vi "isBrushSet.vi"(8 "Error In":errorcluster, 9 "colorRole":T1 items=["WindowText", "Button", "Light", "Midlight", "Dark", "Mid", "Text", "BrightText", "ButtonText", "Base", "Window", "Shadow", "Highlight", "HighlightedText", "Link", "LinkVisited", "AlternateBase", "NoRole", "ToolTipBase", "ToolTipText", "PlaceholderText"], 10 "colorGroup":T2 items=["Active"=0, "Disabled"=1, "Inactive"=2, "All"=5], 11 "QPalette In":refnum<class "QPalette.lvclass">) -> (0 "Error Out":errorcluster, 2 "Value":bool, 3 "QPalette Out":refnum<class "QPalette.lvclass">)   [LabVIEW 2014, in "QPalette.lvclass"]
doc: "LabVIEW-specific documentation is not yet available. See <b>https://doc.qt.io/qt-5/qpalette.html#isBrushSet</b>"
uses:
  QPalette.lvclass
  ColorGroup.ctl
  ColorRole.ctl
  LQ Core/LQSerialData/LQSerialData.lvclass/LQSerialData.ctl
  LQ Core/LQ Core.lvlib
  LQ Core/LQSerialData/LQSerialData.lvclass
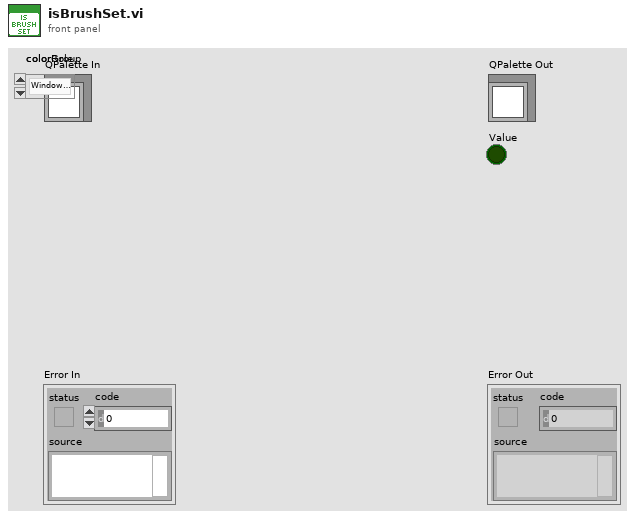
[diagram p1: front panel]
types:
  T1 = typedef "QPalette.lvclass/ColorRole.ctl" = i32
  T2 = typedef "QPalette.lvclass/ColorGroup.ctl" = i32
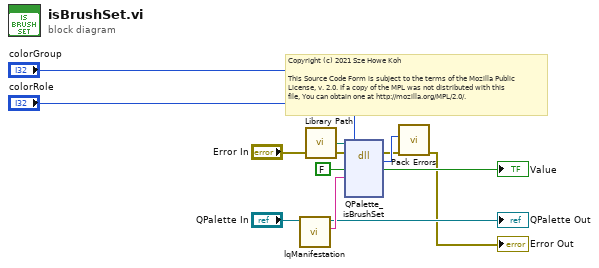
[diagram p0: block diagram]
diagram:
  # "Copyright (c) 2021 Sze Howe Koh\n\nThis Source Code Form is subject to the terms of the Mozilla Public\nLicense, v. 2.0. If a copy of the MPL was not distributed with this\nfile, You can obtain one at http://mozilla.org/MPL/2.0/."
  n1 = call "lqManifestation.vi"("LQSerialData in"="QPalette In") -> ("Manifestation"=w9:string, "LQSerialData out"=→"QPalette Out":refnum<class "QPalette.lvclass">)  [unwired: 9 in]
  n2 = call "Library Path.vi"() -> ("Library Path"=w6:path)
  n3 = dll-call lib="?" fn="QPalette_isBrushSet"(path in=w6, error in="Error In", "_retVal"=FALSE, "_instance"=w9, "colorGroup"="colorGroup", "colorRole"="colorRole") -> (error out=w4:errorcluster, w5:i32, "_retVal"=→"Value":bool)  [unwired: 4 in, 1 out]
  n4 = call "Pack Errors.vi"("Error In"=w4, "Error Code"=w5) -> ("Error Out"=→"Error Out":errorcluster)  [unwired: 9 in]
